vi "Relink to PPL.vi"(11 "VI in":refnum<vi>) -> ()   [LabVIEW 2015, in "Message Maker.lvclass"]
uses:
  Message Maker.lvclass
  <vilib>/Utility/traverseref.llb/TRef TravTarget.ctl
  <vilib>/Utility/traverseref.llb/VI Scripting - Traverse.lvlib
  <vilib>/Utility/VariantDataType/VariantType.lvlib
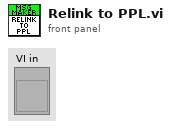
[diagram p1: front panel]
types:
  T1 = typedef "TRef TravTarget.ctl" = enum16{"FP", "BD", "Other"}
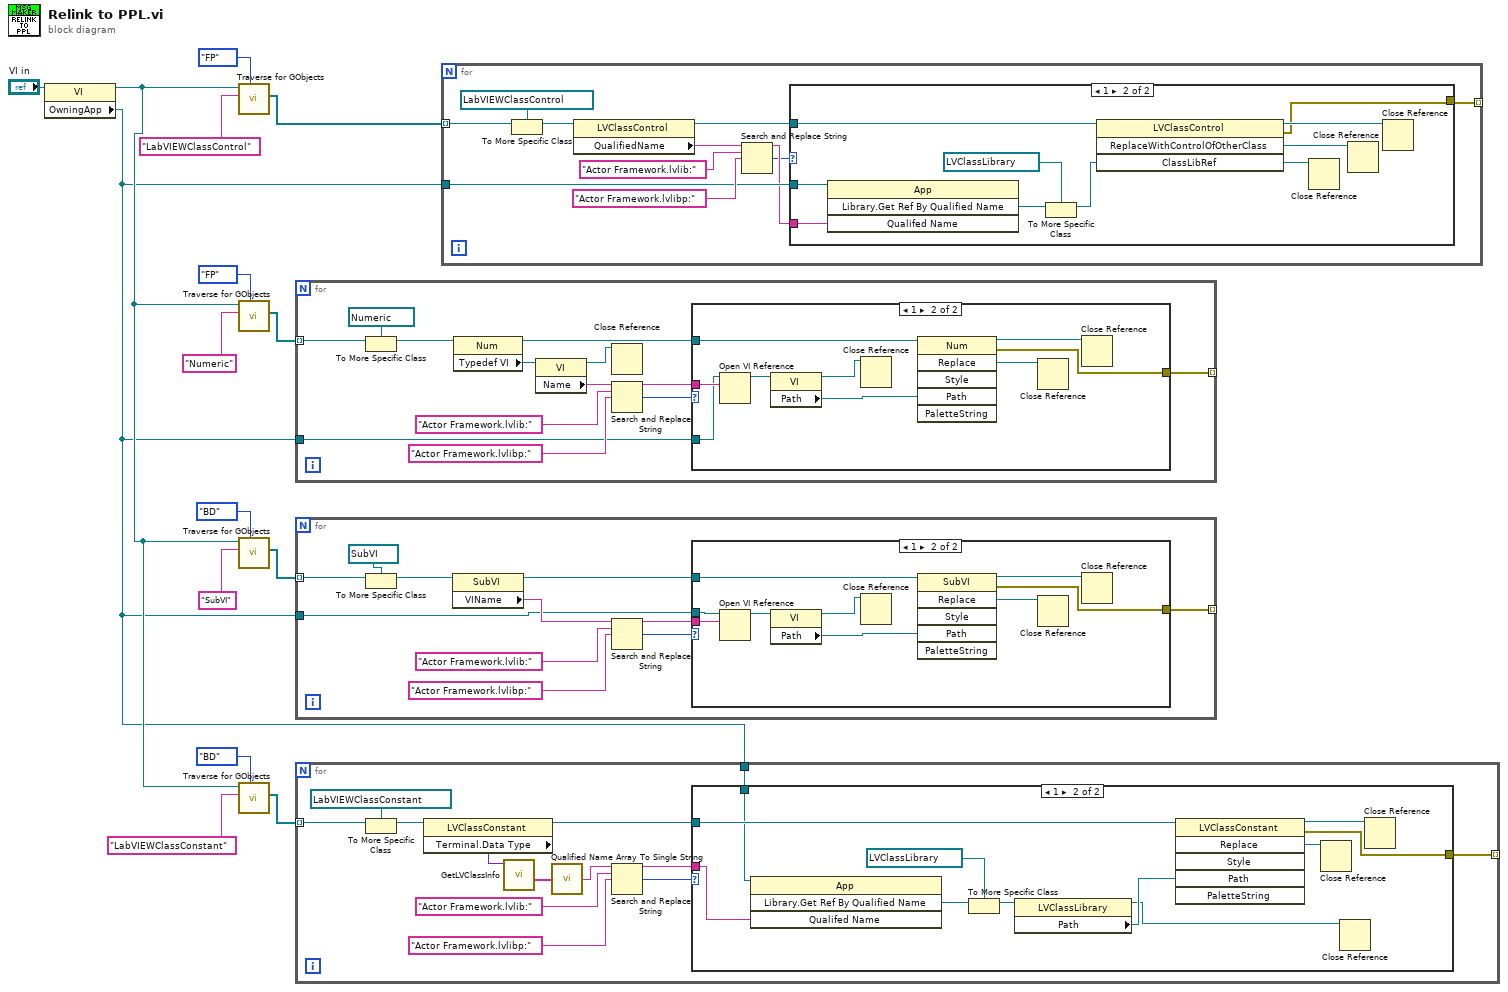
[diagram p0: block diagram]
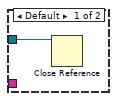
[diagram p2: hidden frame]
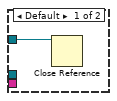
[diagram p3: hidden frame]
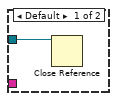
[diagram p4: hidden frame]
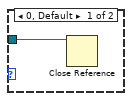
[diagram p5: hidden frame]
diagram:
  n1 = property class="VI"(reference="VI in") -> (reference out=w2:refnum<vi>, "OwningApp"=w1:refnum<vi>)  [unwired: 1 in, 1 out]
  n2 = call <vilib>:"Traverse for GObjects.vi"("Traverse Target"=TRef_TravTarget."FP", "Class Name"="LabVIEWClassControl", "VI Refnum"=w2) -> ("References"=w14:refnum<vi>[])  [unwired: 5 in, 3 out]
  n3 = call <vilib>:"Traverse for GObjects.vi"("Traverse Target"=TRef_TravTarget."FP", "Class Name"="Numeric", "VI Refnum"=w2) -> ("References"=w9:refnum<vi>[])  [unwired: 5 in, 3 out]
  n4 = call <vilib>:"Traverse for GObjects.vi"("Traverse Target"=TRef_TravTarget."BD", "Class Name"="SubVI", "VI Refnum"=w2) -> ("References"=w8:refnum<vi>[])  [unwired: 5 in, 3 out]
  n5 = call <vilib>:"Traverse for GObjects.vi"("Traverse Target"=TRef_TravTarget."BD", "Class Name"="LabVIEWClassConstant", "VI Refnum"=w2) -> ("References"=w3:refnum<vi>[])  [unwired: 5 in, 3 out]
  n6 = for {
    tunnel: w9 -> [w27] mode=indexing
    tunnel: [w17] -> _ mode=indexing
    tunnel: w1 -> [w16]
    n7 = To More Specific Class(target class=refnum<vi> refnum ("reference"), reference=w27) -> (specific class reference=w26:refnum<vi>)  [unwired: 1 in, 1 out]
    n8 = property class="Num"(reference=w26) -> (reference out=w20:refnum<vi>, "Typedef VI"=w25:refnum<vi>)  [unwired: 1 in, 1 out]
    n9 = property class="VI"(reference=w25) -> (reference out=w18:refnum<vi>, "Name"=w24:string)  [unwired: 1 in, 1 out]
    n10 = Close Reference(reference=w18) -> ()  [unwired: 1 in, 1 out]
    n11 = Search and Replace String(input string=w24, search string="Actor Framework.lvlib:", replace string="Actor Framework.lvlibp:" ("search string")) -> (result string=w19:string, number of replacements=w21:i32)  [unwired: 5 in, 2 out]
    n12 = case shown="1" w21 {
      tunnel: w20 -> [w29 w38]
      tunnel: w19 -> [_ w37]
      tunnel: [_ w31] -> w17
      tunnel: w16 -> [_ w30]
      frame Default {
        n13 = Close Reference(reference=w29) -> ()  [unwired: 1 in, 1 out]
      }
      frame 1 {
        n14 = Open VI Reference(application reference (local)=w30, vi path=w37) -> (vi reference=w36:refnum<vi>)  [unwired: 4 in, 1 out]
        n15 = property class="VI"(reference=w36) -> (reference out=w34:refnum<vi>, "Path"=w35:path)  [unwired: 1 in, 1 out]
        n16 = Close Reference(reference=w34) -> ()  [unwired: 1 in, 1 out]
        n17 = invoke class="Num" method="Replace"(reference=w38, "Path"=w35) -> (reference out=w32:refnum<vi>, error out=w31:errorcluster, "Replace"=w33:refnum<vi>)  [unwired: 4 in, 3 out]
        n18 = Close Reference(reference=w33) -> ()  [unwired: 1 in, 1 out]
        n19 = Close Reference(reference=w32) -> ()  [unwired: 1 in, 1 out]
      }
    }
  }
  n20 = for {
    tunnel: w8 -> [w48] mode=indexing
    tunnel: [w41] -> _ mode=indexing
    tunnel: w1 -> [w39]
    n21 = To More Specific Class(target class=refnum<vi> refnum ("reference"), reference=w48) -> (specific class reference=w47:refnum<vi>)  [unwired: 1 in, 1 out]
    n22 = property class="SubVI"(reference=w47) -> (reference out=w43:refnum<vi>, "VIName"=w40:string)  [unwired: 1 in, 1 out]
    n23 = Search and Replace String(input string=w40, search string="Actor Framework.lvlib:", replace string="Actor Framework.lvlibp:" ("search string")) -> (result string=w42:string, number of replacements=w44:i32)  [unwired: 5 in, 2 out]
    n24 = case shown="1" w44 {
      tunnel: w43 -> [w50 w59]
      tunnel: w42 -> [_ w58]
      tunnel: [_ w52] -> w41
      tunnel: w39 -> [_ w51]
      frame Default {
        n25 = Close Reference(reference=w50) -> ()  [unwired: 1 in, 1 out]
      }
      frame 1 {
        n26 = Open VI Reference(application reference (local)=w51, vi path=w58) -> (vi reference=w57:refnum<vi>)  [unwired: 4 in, 1 out]
        n27 = property class="VI"(reference=w57) -> (reference out=w55:refnum<vi>, "Path"=w56:path)  [unwired: 1 in, 1 out]
        n28 = Close Reference(reference=w55) -> ()  [unwired: 1 in, 1 out]
        n29 = invoke class="SubVI" method="Replace"(reference=w59, "Path"=w56) -> (reference out=w53:refnum<vi>, error out=w52:errorcluster, "Replace"=w54:refnum<vi>)  [unwired: 4 in, 3 out]
        n30 = Close Reference(reference=w54) -> ()  [unwired: 1 in, 1 out]
        n31 = Close Reference(reference=w53) -> ()  [unwired: 1 in, 1 out]
      }
    }
  }
  n32 = for {
    tunnel: w3 -> [w71] mode=indexing
    tunnel: [w64] -> _ mode=indexing
    tunnel: w1 -> [w60]
    n33 = To More Specific Class(target class=refnum<vi> refnum ("reference"), reference=w71) -> (specific class reference=w70:refnum<vi>)  [unwired: 1 in, 1 out]
    n34 = property class="LVClassConstant"(reference=w70) -> (reference out=w66:refnum<vi>, "Terminal.Data Type"=w62:variant)  [unwired: 1 in, 1 out]
    n35 = call <vilib>:"GetLVClassInfo.vi"("Variant"=w62) -> ("Fully Qualified LV Class Name"=w63:string[])  [unwired: 8 in, 2 out]
    n36 = call <vilib>:"Qualified Name Array To Single String.vi"("Fully Qualified Array"=w63) -> ("Fully Qualified String"=w61:string)
    n37 = Search and Replace String(input string=w61, search string="Actor Framework.lvlib:", replace string="Actor Framework.lvlibp:" ("search string")) -> (result string=w65:string, number of replacements=w67:i32)  [unwired: 5 in, 2 out]
    n38 = case shown="1" w67 {
      tunnel: w66 -> [w73 w84]
      tunnel: w65 -> [_ w78]
      tunnel: [_ w81] -> w64
      tunnel: w60 -> [_ w77]
      frame Default {
        n39 = Close Reference(reference=w73) -> ()  [unwired: 1 in, 1 out]
      }
      frame 1 {
        n40 = invoke class="App" method="Library.Get Ref By Qualified Name"(reference=w77, "Qualifed Name"=w78) -> ("Library.Get Ref By Qualified Name"=w80:refnum<vi>)  [unwired: 2 in, 3 out]
        n41 = To More Specific Class(target class=refnum<vi> refnum ("ReplacementClassLibRef"), reference=w80) -> (specific class reference=w76:refnum<vi>)  [unwired: 1 in, 1 out]
        n42 = property class="LVClassLibrary"(reference=w76) -> (reference out=w74:refnum<vi>, "Path"=w75:path)  [unwired: 1 in, 1 out]
        n43 = invoke class="LVClassConstant" method="Replace"(reference=w84, "Path"=w75) -> (reference out=w82:refnum<vi>, error out=w81:errorcluster, "Replace"=w83:refnum<vi>)  [unwired: 4 in, 3 out]
        n44 = Close Reference(reference=w83) -> ()  [unwired: 1 in, 1 out]
        n45 = Close Reference(reference=w74) -> ()  [unwired: 1 in, 1 out]
        n46 = Close Reference(reference=w82) -> ()  [unwired: 1 in, 1 out]
      }
    }
  }
  n47 = for {
    tunnel: w14 -> [w94] mode=indexing
    tunnel: w1 -> [w88]
    tunnel: [w86] -> _ mode=indexing
    n48 = To More Specific Class(target class=refnum<vi> refnum ("reference"), reference=w94) -> (specific class reference=w93:refnum<vi>)  [unwired: 1 in, 1 out]
    n49 = property class="LVClassControl"(reference=w93) -> (reference out=w92:refnum<vi>, "QualifiedName"=w91:string)  [unwired: 1 in, 1 out]
    n50 = Search and Replace String(input string=w91, search string="Actor Framework.lvlib:", replace string="Actor Framework.lvlibp:" ("search string")) -> (result string=w87:string, number of replacements=w85:i32)  [unwired: 5 in, 2 out]
    n51 = case shown="1" w85 {
      tunnel: w92 -> [w96 w106]
      tunnel: w88 -> [_ w105]
      tunnel: w87 -> [_ w101]
      tunnel: [_ w97] -> w86
      frame 0, Default {
        n52 = Close Reference(reference=w96) -> ()  [unwired: 1 in, 1 out]
      }
      frame 1 {
        n53 = invoke class="App" method="Library.Get Ref By Qualified Name"(reference=w105, "Qualifed Name"=w101) -> ("Library.Get Ref By Qualified Name"=w104:refnum<vi>)  [unwired: 2 in, 3 out]
        n54 = To More Specific Class(target class=refnum<vi> refnum ("ReplacementClassLibRef"), reference=w104) -> (specific class reference=w102:refnum<vi>)  [unwired: 1 in, 1 out]
        n55 = invoke class="LVClassControl" method="ReplaceWithControlOfOtherClass"(reference=w106, "ClassLibRef"=w102) -> (reference out=w98:refnum<vi>, error out=w97:errorcluster, "ReplaceWithControlOfOtherClass"=w100:refnum<vi>, "ClassLibRef"=w99:refnum<vi>)  [unwired: 2 in]
        n56 = Close Reference(reference=w99) -> ()  [unwired: 1 in, 1 out]
        n57 = Close Reference(reference=w100) -> ()  [unwired: 1 in, 1 out]
        n58 = Close Reference(reference=w98) -> ()  [unwired: 1 in, 1 out]
      }
    }
  }
